vi "Persist Entity.vi"(8 "error in (no error)":errorcluster, 10 "Conditum:Entity":refnum<class "Entity.lvclass">, 11 "Entity Manager in":refnum<class "Entity Manager.lvclass">) -> (0 "error out":errorcluster, 3 "Entity Manager out":refnum<class "Entity Manager.lvclass">)   [LabVIEW 2020, in "Conditum.lvlib" / "Entity Manager.lvclass"]
uses:
  Entity Manager.lvclass
  Database Platform/Database Platform.lvclass
  Entity/Entity.lvclass
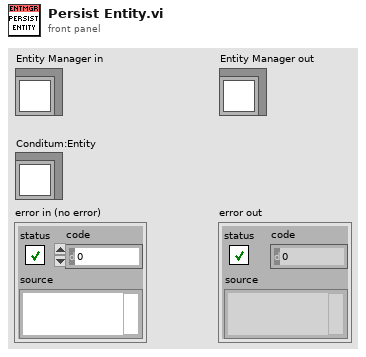
[diagram p1: front panel]
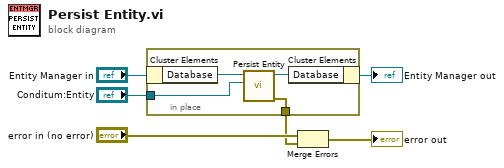
[diagram p0: block diagram]
diagram:
  n1 = in-place {
    in-place-border: "Conditum:Entity" -> [w9]
    in-place-border: [w7] -> w1
    n2 = in-place-cluster #1("Entity Manager in") -> ("Database"=w10:refnum<class "Database Platform.lvclass">)
    n3 = call-dynamic "Persist Entity.vi"("Conditum:Entity"=w9, "Database in"=w10) -> ("error out"=w7:errorcluster, "Database out"=w8:refnum<class "Database Platform.lvclass">)  [unwired: 8 in]
    n4 = in-place-cluster #1("Database"=w8) -> (→"Entity Manager out":refnum<class "Entity Manager.lvclass">)
  }
  n5 = Merge Errors("error in (no error)", w1) -> (→"error out":errorcluster)
